vi "Close Instrument.vi"(8 "error in (no error)":errorcluster, 11 "Simulated Scope.lvclass in":refnum<class "Simulated Scope.lvclass">) -> (0 "error out":errorcluster, 3 "Simulated Scope.lvclass out":refnum<class "Simulated Scope.lvclass">)   [LabVIEW 2010, in "Simulated Scope.lvclass"]
uses:
  Simulated Scope.lvclass
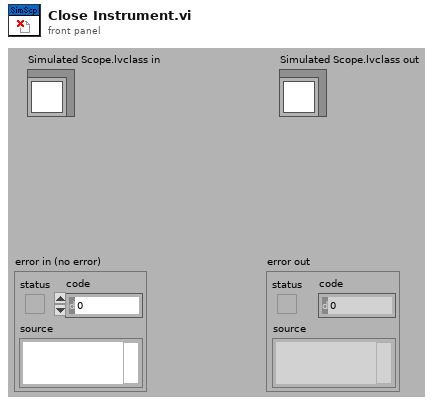
[diagram p1: front panel]
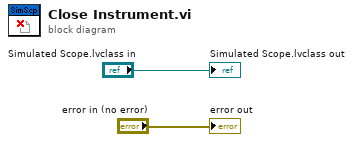
[diagram p0: block diagram]
diagram:
  "error out" <- "error in (no error)"
  "Simulated Scope.lvclass out" <- "Simulated Scope.lvclass in"
